vi "tmpStatistic.vi"(11 "My Std":dbl) -> (0 "Array":u64[][](array[numeric]))   [LabVIEW 2023]
uses:
  <vilib>/Analysis/NI_AALBase.lvlib
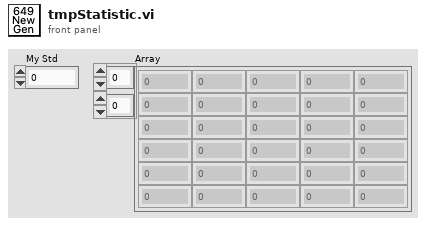
[diagram p1: front panel]
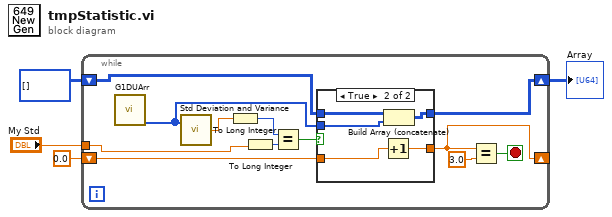
[diagram p0: block diagram]
diagram:
  n1 = while {
    shift-right: [w8] -> w3
    shift-left: u64[][] [] -> [w13]
    shift-right: [w11] -> _
    shift-left: 0.0 -> [w12]
    tunnel: "My Std" -> [w5]
    stop <- w9 stop-if-true
    n2 = call "G1DUArr.vi"() -> ("1D UArr"=w14:u64[])  [unwired: 11 in]
    n3 = call <vilib>:"Std Deviation and Variance.vi"("X"=w14) -> ("standard deviation"=w16:dbl)  [unwired: 1 in, 2 out]
    n4 = To Long Integer(number=w16) -> (32bit integer=w7:i32)
    n5 = To Long Integer(number=w5) -> (32bit integer=w6:i32)
    n6 = Equal?(x=w7, y=w6) -> (x = y?=w15:bool)
    n7 = case shown="True" w15 {
      tunnel: w14 -> [_ w23]
      tunnel: [w18 w22] -> w8
      tunnel: w13 -> [w18 w21]
      tunnel: [w17 w20] -> w11
      tunnel: w12 -> [w17 w19]
      frame False {
      }
      frame True {
        n8 = Increment(x=w19) -> (x+1=w20:dbl)
        n9 = Build Array (concatenate)(w21, w23) -> (w22:u64[][])
      }
    }
    n10 = Equal?(x=w11, y=3.0) -> (x = y?=w9:bool)
  }
  "Array" <- w3
